vi "Get Cargo Capacity.vi"(8 "error in":errorcluster, 11 "truck":refnum<class "Truck.lvclass">) -> (0 "error out":errorcluster, 2 "cargo capacity":dbl)   [LabVIEW 2012, in "Truck.lvclass"]
doc: "This VI is an example of an override member VI. It returns the cargo capacity for the truck."
uses:
  Truck.lvclass
  Vehicle/Vehicle.lvclass
  Truck.lvclass/Truck.ctl
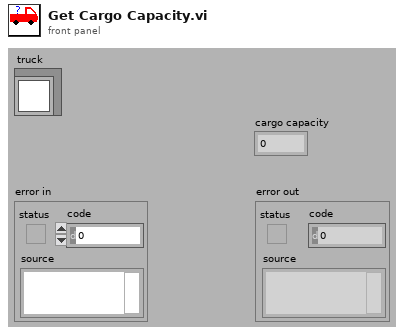
[diagram p1: front panel]
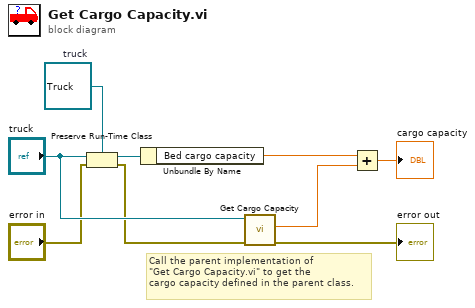
[diagram p0: block diagram]
diagram:
  w3 = refnum<class "Truck.lvclass"> refnum  # truck
  # "Call the parent implementation of\n\"Get Cargo Capacity.vi\" to get the\ncargo capacity defined in the parent class."
  n1 = Preserve Run-Time Class(object in="truck", error in="error in", 2:w3) -> (object out=w4:refnum<class "Truck.lvclass">, error out=w1:errorcluster)
  n2 = Unbundle By Name(w4) -> ("Bed cargo capacity"=w7:dbl)
  n3 = call-parent "Get Cargo Capacity.vi"("error in"=w1, "vehicle"="truck") -> ("error out"=→"error out":errorcluster, "cargo capacity"=w6:dbl)  [unwired: 8 in]
  n4 = Add(x=w7, y=w6) -> (x+y=→"cargo capacity":dbl)
